vi "Create.vi"(10 "API":refnum<class "API.lvclass">) -> (3 "ApiValue out":refnum<class "ApiValue.lvclass">)   [LabVIEW 2020, in "Volatus.lvlib" / "ApiValue.lvclass"]
uses:
  ApiValue.lvclass
  ApiValue.lvclass/ApiValue.ctl
  API/API.lvclass
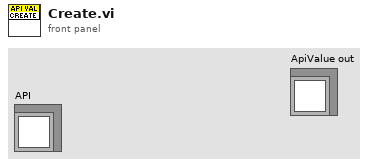
[diagram p1: front panel]
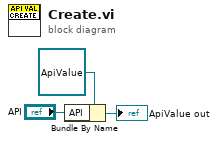
[diagram p0: block diagram]
diagram:
  n1 = Bundle By Name(cluster=refnum<class "ApiValue.lvclass"> refnum ("ApiValue in"), "API"="API") -> (→"ApiValue out":refnum<class "ApiValue.lvclass">)
